vi "Write Encryption Type.vi"(8 "error in (no error)":errorcluster, 10 "Encryption Type":refnum<class "iEncryption.lvclass">, 11 "User Configuration Manager in":refnum<class "User Configuration Manager.lvclass">) -> (0 "error out":errorcluster, 3 "User Configuration Manager out":refnum<class "User Configuration Manager.lvclass">)   [LabVIEW 2019, in "User Configuration Manager.lvlib" / "User Configuration Manager.lvclass"]
uses:
  <vilib>/gpm_packages/@cs/user-manager/Source/User Configuration Manager/User Configuration Manager.lvclass
  <vilib>/gpm_packages/@cs/user-manager/Source/iEncryption/iEncryption.lvclass
  <vilib>/gpm_packages/@cs/user-manager/Source/User Configuration Manager/User Configuration Manager.lvclass/User Configuration Manager.ctl
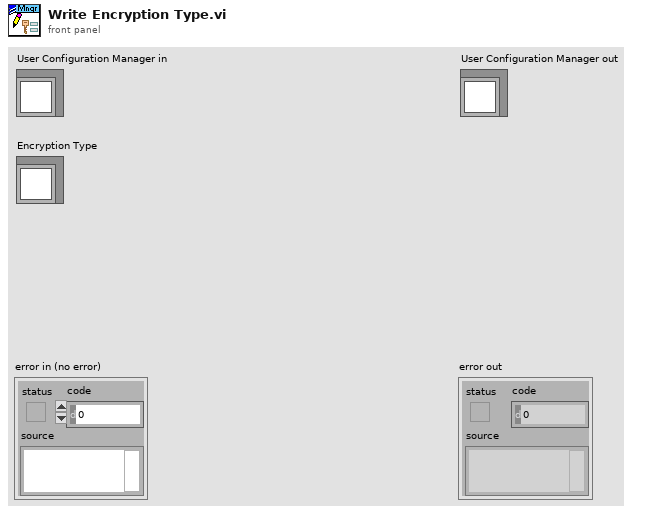
[diagram p1: front panel]
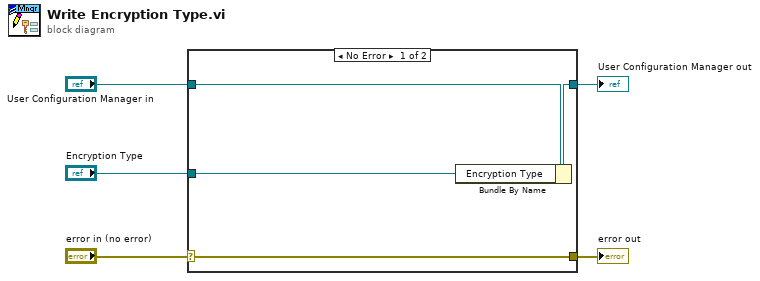
[diagram p0: block diagram]
diagram:
  n1 = case shown="No Error" "error in (no error)" {
    selector: "error in (no error)" -> [w9 w10]
    tunnel: [w9 w10] -> w4
    tunnel: [w7 w11] -> w2
    tunnel: "User Configuration Manager in" -> [w8 w11]
    tunnel: "Encryption Type" -> [w6 _]
    frame No Error {
      n2 = Bundle By Name(cluster=w8, "Encryption Type"=w6) -> (w7:refnum<class "User Configuration Manager.lvclass">)
    }
    frame Error {
    }
  }
  "error out" <- w4
  "User Configuration Manager out" <- w2
